vi "FGV PC Network Settings.vi"(8 "error in (no error)":errorcluster, 10 "PC Network Settings In":T1={"TCP/IP Address"="10.0.0.101", "TCP/IP Port"=55555, "UDP/IP Address"="0.0.0.0", "UDP/IP Port"=55555, "USB Address"="172.22.11.2", "USB Port"=55555, "NS Reader Name"="DAA_Receiver", "NS Writer URL"="//10.0.0.101/DAA_Transmitter"}, 11 "Function":enum16{"Initialize", "Set State", "Get State"}(ring)) -> (0 "error out":errorcluster, 3 "PC Network Settings Out":T1={"TCP/IP Address"="10.0.0.101", "TCP/IP Port"=55555, "UDP/IP Address"="0.0.0.0", "UDP/IP Port"=55555, "USB Address"="172.22.11.2", "USB Port"=55555, "NS Reader Name"="DAA_Receiver", "NS Writer URL"="//10.0.0.101/DAA_Transmitter"})   [LabVIEW 2020]
uses:
  Type Definitions/PC Network Settings.ctl
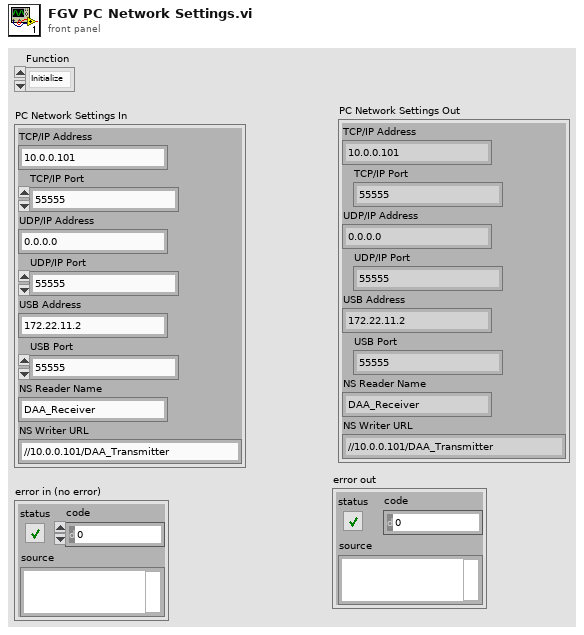
[diagram p1: front panel]
types:
  T1 = typedef "PC Network Settings.ctl" = cluster{"TCP/IP Address":string, "TCP/IP Port":u16, "UDP/IP Address":string, "UDP/IP Port":u16, "USB Address":string, "USB Port":u16, "NS Reader Name":string, "NS Writer URL":string}
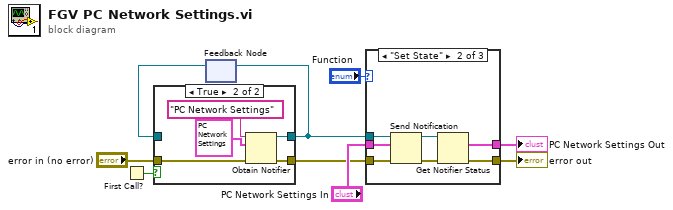
[diagram p0: block diagram]
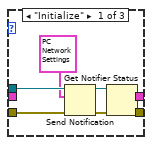
[diagram p3: hidden frame]
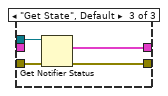
[diagram p4: hidden frame]
diagram:
  n1 = First Call?() -> (First Call?: T/F=w4:bool)
  n2 = feedback #1() -> (w2:refnum<notifier>)  [unwired: 1 in]
  n3 = case shown="True" w4 {
    tunnel: [w11 w15] -> w3
    tunnel: w2 -> [w11 _]
    tunnel: [w10 w14] -> w5
    tunnel: "error in (no error)" -> [w10 w13]
    frame False {
    }
    frame True {
      n4 = Obtain Notifier(name (unnamed)="PC Network Settings", notification data type=T1 {"TCP/IP Address"="10.0.0.101", "TCP/IP Port"=55555, "UDP/IP Address"="0.0.0.0", "UDP/IP Port"=55556, "USB Address"="172.22.11.2", "USB Port"=55557, "NS Reader Name"="DAA_Receiver", "NS Writer URL"="//10.0.0.101/DAA_Transmitter"}, error in (no error)=w13) -> (notifier out=w15:refnum<notifier>, error out=w14:errorcluster)  [unwired: 1 in, 1 out]
    }
  }
  n5 = feedback-in #1(w3) -> ()
  n6 = case shown="\"Set State\"" "Function" {
    tunnel: w3 -> [w23 w30 w33]
    tunnel: [w21 w28 w34] -> w9
    tunnel: w5 -> [w20 w27 w32]
    tunnel: [w18 w25 w31] -> w7
    tunnel: "PC Network Settings In" -> [_ w24 _]
    frame "Initialize" {
      n7 = Send Notification(notification=T1 {"TCP/IP Address"="10.0.0.101", "TCP/IP Port"=55555, "UDP/IP Address"="0.0.0.0", "UDP/IP Port"=55556, "USB Address"="172.22.11.2", "USB Port"=55557, "NS Reader Name"="DAA_Receiver", "NS Writer URL"="//10.0.0.101/DAA_Transmitter"}, notifier=w23, error in (no error)=w20) -> (notifier out=w22:refnum<notifier>, error out=w19:errorcluster)
      n8 = Get Notifier Status(notifier=w22, error in (no error)=w19) -> (current notification=w21:T1, error out=w18:errorcluster)  [unwired: 3 out]
    }
    frame "Set State" {
      n9 = Send Notification(notification=w24, notifier=w30, error in (no error)=w27) -> (notifier out=w29:refnum<notifier>, error out=w26:errorcluster)
      n10 = Get Notifier Status(notifier=w29, error in (no error)=w26) -> (current notification=w28:T1, error out=w25:errorcluster)  [unwired: 3 out]
    }
    frame "Get State", Default {
      n11 = Get Notifier Status(notifier=w33, error in (no error)=w32) -> (current notification=w34:T1, error out=w31:errorcluster)  [unwired: 3 out]
    }
  }
  "error out" <- w7
  "PC Network Settings Out" <- w9
